vi "WriteIQ_int16.vi"(8 "error in (no error)":errorcluster, 9 "dt":dbl=1.0, 10 "data":i16[](array[numeric]), 11 "reference in":refnum<class "IQBurst_memo.lvclass">) -> (0 "error out":errorcluster, 3 "reference out":refnum<class "IQBurst_memo.lvclass">)   [LabVIEW 2019, in "IQBurst_memo.lvclass"]
doc: "Writes IQ data as I16 waveform"
uses:
  IQBurst_memo.lvclass
  C:/Barkhausen mmWave radar/Development/LV/Barkhausen mmWave hardware control/Host/SubVIs/mmWave data_class/mmWave data.lvclass
  mmWave data_class/mmWave data.lvclass
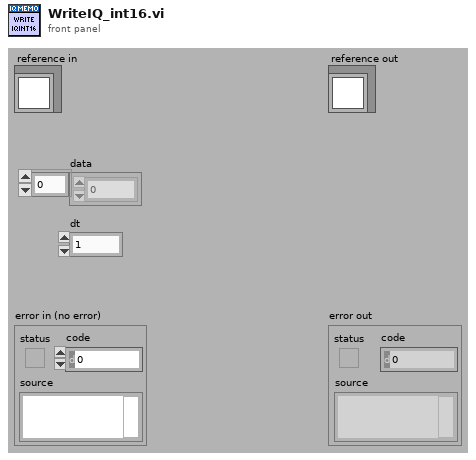
[diagram p1: front panel]
types:
  T1 = typedef "IQBurst_memo.lvclass/ObjectAttributesRef.ctl" = refnum<data-value>
  T2 = typedef "mmWave data.lvclass/ObjectAttributesRef.ctl" = refnum<data-value>
  T3 = typedef "mmWave data.lvclass/ObjectAttributes.ctl" = cluster{"MyAttribute":dbl, "size":i32}
  T4 = typedef "IQBurst_memo.lvclass/ObjectAttributes.ctl" = cluster{"IQ data":i16[], "dt":dbl}
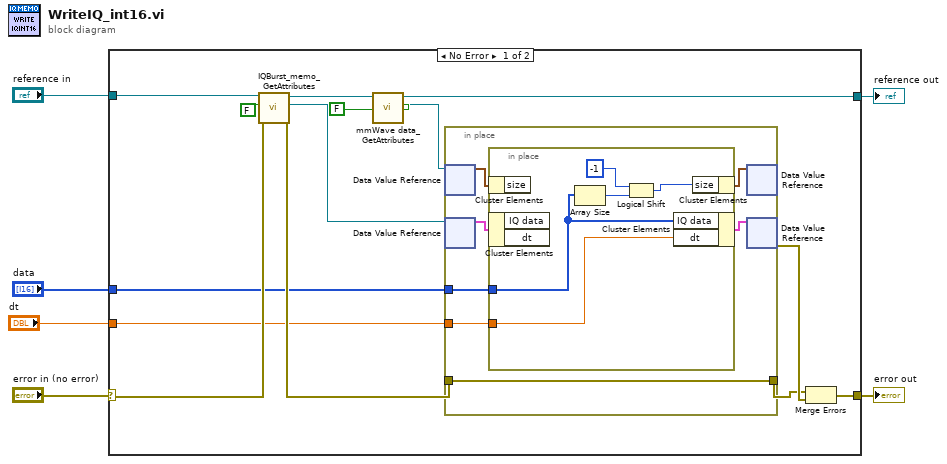
[diagram p0: block diagram]
diagram:
  n1 = case shown="No Error" "error in (no error)" {
    selector: "error in (no error)" -> [w15 w34]
    tunnel: [w20 w34] -> w5
    tunnel: [w9 w33] -> w3
    tunnel: "reference in" -> [w17 w33]
    tunnel: "data" -> [w11 _]
    tunnel: "dt" -> [w10 _]
    frame No Error {
      n2 = call "IQBurst_memo_GetAttributes.vi"("error in (no error)"=w15, "return data? (T)"=FALSE, "reference in"=w17) -> ("error out"=w14:errorcluster, "attributes ref"=w12:T1, "reference out"=w13:refnum<class "IQBurst_memo.lvclass">)  [unwired: 5 in, 1 out]
      n3 = call "mmWave data_GetAttributes.vi"("return data? (T)"=FALSE, "reference in"=w13) -> ("attributes ref"=w7:T2, "reference out"=w9:refnum<class "IQBurst_memo.lvclass">)  [unwired: 6 in, 2 out]
      n4 = in-place {
        in-place-border: w14 -> [w25]
        in-place-border: [w25] -> w18
        in-place-border: w11 -> [w24]
        in-place-border: w10 -> [w23]
        n5 = in-place-dvr #1(w7) -> (w22:T3)  [unwired: 1 out]
        n6 = in-place-dvr #2(w12) -> (w26:T4)  [unwired: 1 out]
        n7 = in-place {
          in-place-border: w24 -> [w31]
          in-place-border: w23 -> [w32]
          n8 = in-place-cluster #3(w22) -> ()  [unwired: 1 out]
          n9 = in-place-cluster #4(w26) -> ()  [unwired: 2 out]
          n10 = Array Size(array=w31) -> (size(s)=w30:i32)
          n11 = Logical Shift(y=i16 -1, x=w30) -> (x << y=w28:i32)
          n12 = in-place-cluster #4("IQ data"=w31, "dt"=w32) -> (w27:T4)
          n13 = in-place-cluster #3("size"=w28) -> (w21:T3)
        }
        n14 = in-place-dvr #1(w21) -> ()  [unwired: 2 out]
        n15 = in-place-dvr #2(w27) -> (w19:errorcluster)  [unwired: 1 out]
      }
      n16 = Merge Errors(w18, w19) -> (w20:errorcluster)
    }
    frame Error {
    }
  }
  "error out" <- w5
  "reference out" <- w3
